vi "Scale Z values to colors.vi"(6 "Scale":T1=enum."RWB", 8 "error in":errorcluster, 11 "Values":dbl[][](array[numeric])) -> (0 "error out":errorcluster, 2 "Color Table":u32[](array[numeric]), 3 "Colors":u32[][](array[colorbox]))   [LabVIEW 2009]
doc: "This VI normalizes and scales 2-d numeric arrays to a color scale for creating intensity plots. The VI is capable of generating a number of different scales, defined by the Scale input. The VI returns a 2-d array of colors representing the magnitude of the original data points upon the seleted scale. The VI also returns a 256 element array of colors which represent the scale used. The color table is useful for creating a legend for the data.\n\nTo add additional scales to this VI, add an item to the Scales typedef and add a case to the Z Value to Color.vi containing the formula for the new scale."
uses:
  Controls/Color Scales.ctl
  <vilib>/Analysis/baseanly.llb/Quick Scale 2D.vi
  <vilib>/Analysis/NI_AALBase.lvlib
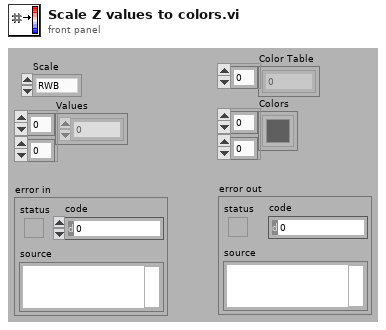
[diagram p1: front panel]
types:
  T1 = typedef "Color Scales.ctl" = enum16{"RGB", "RWB", "BGR", "BWR", "BW", "WB"}
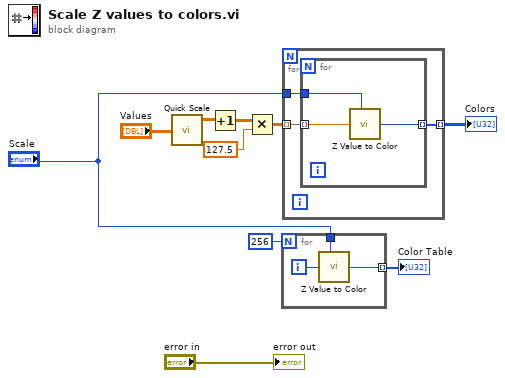
[diagram p0: block diagram]
diagram:
  n1 = call-poly <vilib>:"Quick Scale.vi"("X"="Values") -> ("Yij=Xij/Max|X|"=w3:dbl[][])  [unwired: 2 out]
  n2 = Increment(x=w3) -> (x+1=w2:dbl[][])
  n3 = Multiply ("Multiply.vi")(x=w2, y=127.5) -> (x*y=w8:dbl[][])
  n4 = for {
    N: 256 -> [_]
    tunnel: [w12] -> w5 mode=indexing
    tunnel: "Scale" -> [w11]
    i -> [w13]
    n5 = call "Z Value to Color.vi"("Scale"=w11, "Numeric"=w13) -> ("Color"=w12:u32)  [unwired: 5 in]
  }
  "Color Table" <- w5
  n6 = for {
    tunnel: w8 -> [w16] mode=indexing
    tunnel: [w15] -> w10 mode=indexing
    tunnel: "Scale" -> [w14]
    n7 = for {
      tunnel: w16 -> [w19] mode=indexing
      tunnel: [w18] -> w15 mode=indexing
      tunnel: w14 -> [w17]
      n8 = call "Z Value to Color.vi"("Scale"=w17, "Numeric"=w19) -> ("Color"=w18:u32)  [unwired: 5 in]
    }
  }
  "Colors" <- w10
  "error out" <- "error in"
